vi "Save-As-Default (SubVI) - 12-22-11.vi"(0 "Current VI's Path":path, 5 "Load Settings":bool, 7 "Save Settings":bool, 9 "Save and Exit":bool, 11 "Error Input":errorcluster) -> (15 "Error Output":errorcluster)   [LabVIEW 2011]
panel:
  # "Save As Defaults (SubVI) - Created by Blake Otting - October 2007\nUpdated 12/22/2011"
  # "Connect As Shown \nin Main Program VI"
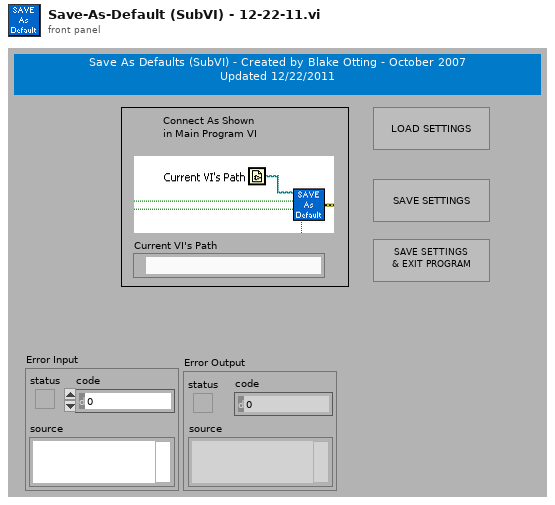
[diagram p1: front panel]
types:
  T1 = enum16{"open", "replace", "create", "open or create", "replace or create", "replace or create with confirmation"}
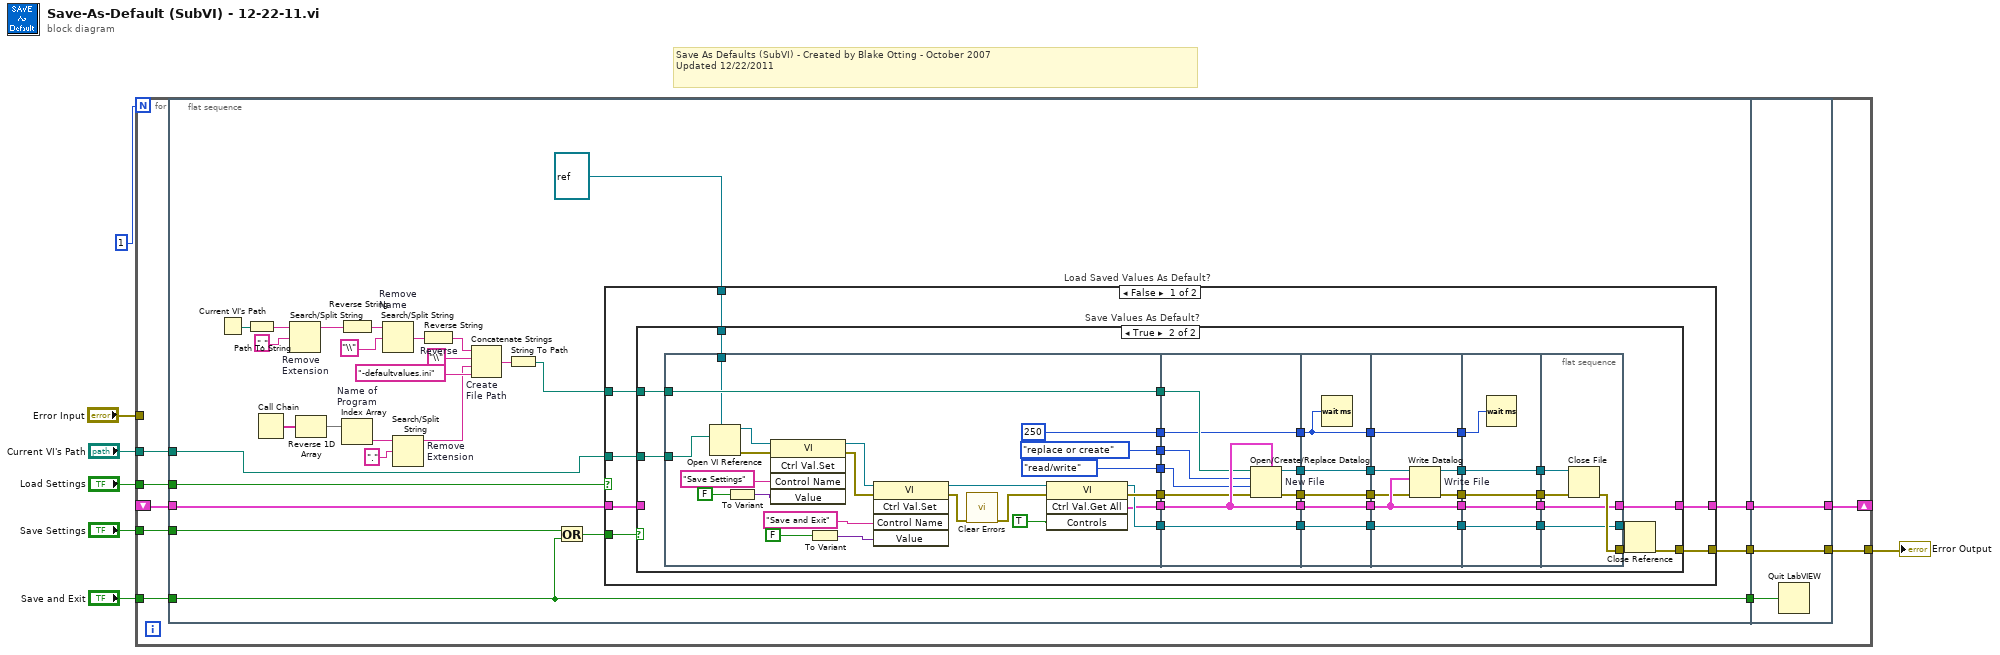
[diagram p0: block diagram]
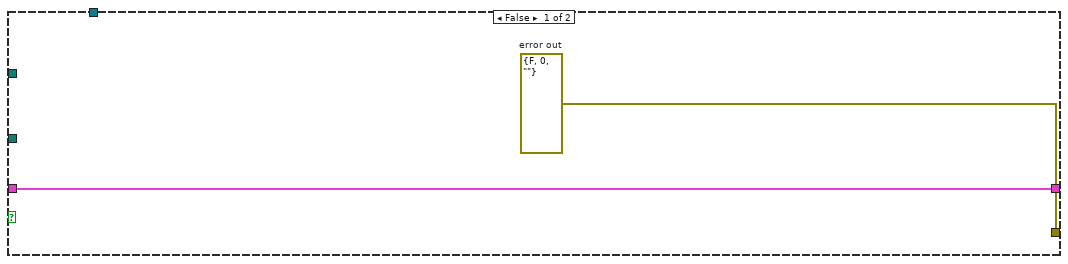
[diagram p2: hidden frame]
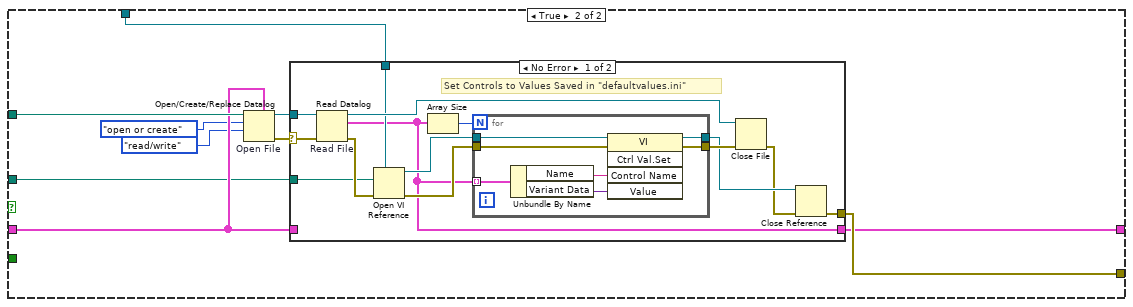
[diagram p3: hidden frame]
diagram:
  # "Save As Defaults (SubVI) - Created by Blake Otting - October 2007\nUpdated 12/22/2011"
  n1 = for {
    N: 1 -> [_]
    shift-right: [w17] -> _
    shift-left: _ -> [w16]
    tunnel: [w15] -> w3
    tunnel: "Save and Exit" -> [w10]
    tunnel: "Load Settings" -> [w9]
    tunnel: "Save Settings" -> [w11]
    tunnel: "Error Input" -> [_]
    tunnel: "Current VI's Path" -> [w8]
    n2 = flat-sequence {
      tunnel: [w42] -> w14
      tunnel: [w40] -> w13
      tunnel: [w39] -> w12
      tunnel: w9 -> [w36]
      tunnel: w10 -> [w39]
      tunnel: w11 -> [w38]
      tunnel: w16 -> [w43]
      tunnel: w8 -> [w19]
      tunnel: [w174] -> w15
      tunnel: [w175] -> w17
      tunnel: w14 -> [w175]
      tunnel: w13 -> [w174]
      tunnel: w12 -> [w173]
      frame #0 {
        n3 = Current VI's Path() -> (path=w18:path)
        n4 = Path To String(path=w18) -> (string=w23:string)
        n5 = Call Chain() -> (call chain=w31:string[])
        n6 = Search/Split String "Remove \nExtension"(string=w23, search string/char (-)=".") -> (substring before match=w24:string)  [unwired: 1 in, 2 out]
        n7 = Reverse 1D Array(array=w31) -> (reversed array=w30:string[])
        n8 = Reverse String ("Reverse")(1:w24) -> (0:w25:string)
        n9 = Index Array "Name of\nProgram"(array=w30) -> (element=w32:string)  [unwired: 1 in]
        n10 = Search/Split String "Remove\nName"(string=w25, search string/char (-)="\\") -> (match + rest of string=w27:string)  [unwired: 1 in, 2 out]
        n11 = Search/Split String "Remove \nExtension"(string=w32, search string/char (-)=".") -> (substring before match=w34:string)  [unwired: 1 in, 2 out]
        n12 = Reverse String "Reverse"(1:w27) -> (0:w28:string)
        n13 = Concatenate Strings "Create\nFile Path"(w28, "\\", w34, "-defaultvalues.ini") -> (w21:string)
        n14 = String To Path(string=w21) -> (path=w20:path)
        n15 = Or(x=w38, y=w39) -> (x .or. y?=w41:bool)
        n16 = case "Load Saved Values As Default?" shown="False" w36 {
          tunnel: [w50 w149] -> w40
          tunnel: w20 -> [w49 w147]
          tunnel: w41 -> [w48 _]
          tunnel: w43 -> [w47 w146]
          tunnel: [w44 w148] -> w42
          tunnel: w19 -> [w46 w144]
          tunnel: refnum<vi> refnum ("Application Reference Input 2") -> [w45 w145]
          frame False {
            n17 = case "Save Values As Default?" shown="True" w48 {
              tunnel: [w51 w85] -> w50
              tunnel: w49 -> [_ w84]
              tunnel: [w52 w83] -> w44
              tunnel: w47 -> [w52 _]
              tunnel: w46 -> [_ w53]
              tunnel: w45 -> [_ w54]
              frame False {
                w51 = errorcluster {"status"=FALSE, "code"=0, "source"=""}  # error out
              }
              frame True {
                n18 = flat-sequence {
                  tunnel: w84 -> [w108]
                  tunnel: [w90] -> w63
                  tunnel: [enum16{"read/write", "read-only", "write-only"}."read/write" ("access (0:read/write)")] -> w62
                  tunnel: [T1."replace or create" ("operation (0:open)")] -> w61
                  tunnel: [w88] -> w60
                  tunnel: [w108] -> w59
                  tunnel: [w89] -> w58
                  tunnel: [u32 250 ("milliseconds to wait")] -> w57
                  tunnel: w54 -> [w92]
                  tunnel: w53 -> [w91]
                  tunnel: [w113] -> w82
                  tunnel: [w112] -> w80
                  tunnel: [w117] -> w78
                  tunnel: [w110] -> w76
                  tunnel: [w109] -> w64
                  tunnel: w63 -> [w116]
                  tunnel: w62 -> [w115]
                  tunnel: w61 -> [w114]
                  tunnel: w60 -> [w117]
                  tunnel: w59 -> [w111]
                  tunnel: w58 -> [w110]
                  tunnel: w57 -> [w109]
                  tunnel: w82 -> [w122]
                  tunnel: [w122] -> w81
                  tunnel: w80 -> [w121]
                  tunnel: [w121] -> w79
                  tunnel: w78 -> [w120]
                  tunnel: [w120] -> w77
                  tunnel: w76 -> [w119]
                  tunnel: [w119] -> w75
                  tunnel: w64 -> [w118]
                  tunnel: [w118] -> w55
                  tunnel: w81 -> [w127]
                  tunnel: w79 -> [w129]
                  tunnel: w77 -> [w128]
                  tunnel: [w128] -> w74
                  tunnel: w75 -> [w126]
                  tunnel: [w126] -> w72
                  tunnel: [w125] -> w70
                  tunnel: [w124] -> w68
                  tunnel: [w123] -> w56
                  tunnel: w55 -> [w123]
                  tunnel: w74 -> [w134]
                  tunnel: [w134] -> w73
                  tunnel: w72 -> [w133]
                  tunnel: [w133] -> w71
                  tunnel: w70 -> [w132]
                  tunnel: [w132] -> w69
                  tunnel: w68 -> [w131]
                  tunnel: [w131] -> w67
                  tunnel: w56 -> [w130]
                  tunnel: [w138] -> w83
                  tunnel: w73 -> [w138]
                  tunnel: [w137] -> w65
                  tunnel: w71 -> [w137]
                  tunnel: w69 -> [w136]
                  tunnel: w67 -> [w135]
                  tunnel: [w139] -> w66
                  frame #0 {
                    n19 = Open VI Reference(type specifier VI Refnum (for type only)=w92, vi path=w91) -> (vi reference=w100:refnum<vi>, error out=w101:errorcluster)  [unwired: 2 in, 2 out]
                    n20 = To Variant(anything=FALSE ("Controls")) -> (Variant=w99:variant)
                    n21 = invoke class="VI" method="Ctrl Val.Set"(reference=w100, error in=w101, "Control Name"="Save Settings", "Value"=w99) -> (reference out=w104:refnum<vi>, error out=w105:errorcluster)  [unwired: 1 in, 3 out]
                    n22 = To Variant(anything=FALSE ("Controls")) -> (Variant=w102:variant)
                    n23 = invoke class="VI" method="Ctrl Val.Set"(reference=w104, error in=w105, "Control Name"="Save and Exit", "Value"=w102) -> (reference out=w107:refnum<vi>, error out=w87:errorcluster)  [unwired: 1 in, 3 out]
                    n24 = call <vilib>:"Clear Errors.vi"("error in (no error)"=w87) -> ("error out"=w86:errorcluster)  [unwired: 6 out]
                    n25 = invoke class="VI" method="Ctrl Val.Get All"(reference=w107, error in=w86, "Controls"=TRUE) -> (reference out=w89:refnum<vi>, error out=w90:errorcluster, "Get All Control Values Variant"=w88:cluster{"Name":string, "Variant Data":variant}[])  [unwired: 1 in, 1 out]
                  }
                  frame #1 {
                    n26 = Open/Create/Replace Datalog "New File"(5:w117, 8:w116, 9:w115, 10:w114, 11:w111) -> (0:w113:errorcluster, 3:w112:refnum<k1>)  [unwired: 2 out]
                  }
                  frame #2 {
                    n27 = Wait (ms)(milliseconds to wait=w118) -> ()  [unwired: 1 out]
                  }
                  frame #3 {
                    n28 = Write Datalog "Write File"(4:w127, 6:w128, 7:w129) -> (0:w125:errorcluster, 3:w124:refnum<k1>)
                  }
                  frame #4 {
                    n29 = Wait (ms)(milliseconds to wait=w130) -> ()  [unwired: 1 out]
                  }
                  frame #5 {
                    n30 = Close File(refnum=w135, error in=w136) -> (error out=w139:errorcluster)  [unwired: 1 out]
                  }
                }
                n31 = Close Reference(reference=w65, error in (no error)=w66) -> (error out=w85:errorcluster)
              }
            }
          }
          frame True {
            n32 = Open/Create/Replace Datalog "Open File"(5:w146, 9:enum16{"read/write", "read-only", "write-only"}."read/write" ("access (0:read/write)"), 10:T1."open or create" ("operation (0:open)"), 11:w147) -> (0:w143:errorcluster, 3:w142:refnum<k1>)  [unwired: 1 in, 2 out]
            n33 = case shown="No Error" w143 {
              selector: w143 -> [w157 w171]
              tunnel: [w161 w171] -> w149
              tunnel: w146 -> [_ w172]
              tunnel: [w150 w172] -> w148
              tunnel: w142 -> [w158 _]
              tunnel: w145 -> [w154 _]
              tunnel: w144 -> [w153 _]
              frame No Error {
                # "Set Controls to Values Saved in \"defaultvalues.ini\""
                n34 = Read Datalog "Read File"(4:w157, 7:w158) -> (0:w155:errorcluster, 2:w150:cluster{"Name":string, "Variant Data":variant}[], 3:w163:refnum<k1>)  [unwired: 1 out]
                n35 = Open VI Reference(type specifier VI Refnum (for type only)=w154, vi path=w153, error in (no error)=w155) -> (vi reference=w156:refnum<vi>, error out=w152:errorcluster)  [unwired: 1 in, 2 out]
                n36 = Array Size(array=w150) -> (size(s)=w151:i32)
                n37 = for {
                  N: w151 -> [_]
                  tunnel: w150 -> [w166] mode=indexing
                  tunnel: w152 -> [w168]
                  tunnel: [w169] -> w162
                  tunnel: w156 -> [w167]
                  tunnel: [w164] -> w160
                  n38 = Unbundle By Name(w166) -> ("Name"=w165:string, "Variant Data"=w170:variant)
                  n39 = invoke class="VI" method="Ctrl Val.Set"(reference=w167, error in=w168, "Control Name"=w165, "Value"=w170) -> (reference out=w164:refnum<vi>, error out=w169:errorcluster)  [unwired: 1 in, 3 out]
                }
                n40 = Close File(refnum=w163, error in=w162) -> (error out=w159:errorcluster)  [unwired: 1 out]
                n41 = Close Reference(reference=w160, error in (no error)=w159) -> (error out=w161:errorcluster)
              }
              frame Error {
                # "\"defaultvalues.ini\" Not Found"
              }
            }
          }
        }
      }
      frame #1 {
        n42 = Quit LabVIEW(quit? (T)=w173) -> ()
      }
    }
  }
  "Error Output" <- w3
